vi "Read Multi Eval Meas Magnitude Error Results.vi"(8 "error in (no error)":errorcluster, 9 "Result Type (Current)":i32(ring) items=["Current"=0, "Average"=1, "Maximum"=4], 10 "Instance (1)":T1=1, 11 "VISA resource name":refnum<visa-resource-name>) -> (0 "error out":errorcluster, 1 "Magnitude Error Results":cluster{"Low Window":dbl, "High Window":dbl}[](array[cluster]) {"High Window" format="%^.3e"; "Low Window" format="%^.3e"}, 2 "Reliability":i32, 3 "VISA resource name out":refnum<visa-resource-name>)   [LabVIEW 2020, in "Rohde&Schwarz CMWXP NR FR1 Measurement.lvlib"]
doc: "Returns the values of the magnitude error bar graphs for the OFDM symbols in the measured slot. The results of the current, average and maximum bar graphs can be retrieved.\n\nThere is one pair of magnitude error values per OFDM symbol, for low and high EVM window position respectively.\n\nAttributes:\nRSCMWXPNRFR1M_ATTR_READ_MULTI_EVAL_MEAS_MAGNITUDE_ERROR_CURRENT_RESULTS\nRSCMWXPNRFR1M_ATTR_READ_MULTI_EVAL_MEAS_MAGNITUDE_ERROR_AVERAGE_RESULTS\nRSCMWXPNRFR1M_ATTR_READ_MULTI_EVAL_MEAS_MAGNITUDE_ERROR_MAXIMUM_RESULTS\n\nRemote-control commands:\nREAD:NRSub:MEAS<i>:MEValuation:MERRor:CURRent?\nREAD:NRSub:MEAS<i>:MEValuation:MERRor:AVERage?\nREAD:NRSub:MEAS<i>:MEValuation:MERRor:MAXimum?"
uses:
  <instrlib>/Rohde&Schwarz CMWXP NR FR1 Measurement/Rohde&Schwarz CMWXP NR FR1 Measurement.lvlib
  <instrlib>/Rohde&Schwarz CMWXP NR FR1 Measurement/Private/_Instance.ctl
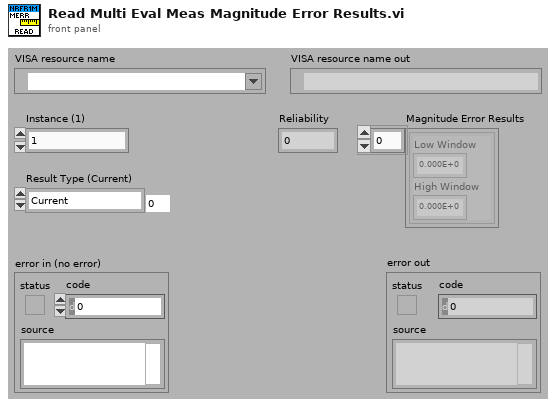
[diagram p1: front panel]
types:
  T1 = typedef "Rohde&Schwarz CMWXP NR FR1 Measurement.lvlib/_Instance.ctl" = i32
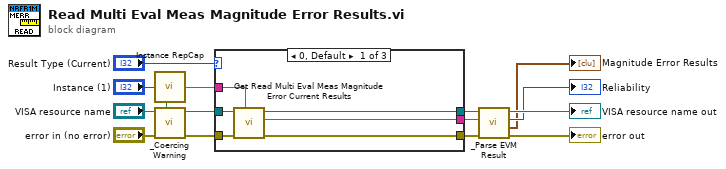
[diagram p0: block diagram]
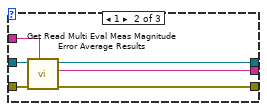
[diagram p2: hidden frame]
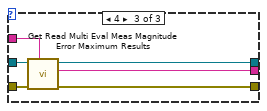
[diagram p3: hidden frame]
diagram:
  n1 = call <instrlib>:"Instance RepCap.vi"("Instance In"="Instance (1)") -> ("In Range?"=w12:bool, "RepCap Identifier Out"=w11:string)  [unwired: 1 in]
  n2 = call <instrlib>:"_Coercing Warning.vi"("In Range?"=w12, "error in (no error)"="error in (no error)", "VISA resource name"="VISA resource name") -> ("error out"=w9:errorcluster, "VISA resource name out"=w10:refnum<visa-resource-name>)  [unwired: 7 in]
  n3 = case shown="0, Default" "Result Type (Current)" {
    tunnel: w11 -> [w21 w27 w33]
    tunnel: w10 -> [w20 w26 w32]
    tunnel: w9 -> [w19 w25 w31]
    tunnel: [w18 w24 w30] -> w5
    tunnel: [w17 w23 w29] -> w6
    tunnel: [w16 w22 w28] -> w7
    frame 0, Default {
      n4 = call "Get Read Multi Eval Meas Magnitude Error Current Results"("Repeated Capabilities"=w21, "error in (no error)"=w19, "instrument handle"=w20) -> ("error out"=w16:errorcluster, "Read Multi Eval Meas Magnitude Error Current Results"=w17:string, "instrument handle out"=w18:refnum<visa-resource-name>)  [unwired: 6 in]
    }
    frame 1 {
      n5 = call "Get Read Multi Eval Meas Magnitude Error Average Results"("Repeated Capabilities"=w27, "error in (no error)"=w25, "instrument handle"=w26) -> ("error out"=w22:errorcluster, "Read Multi Eval Meas Magnitude Error Average Results"=w23:string, "instrument handle out"=w24:refnum<visa-resource-name>)  [unwired: 6 in]
    }
    frame 4 {
      n6 = call "Get Read Multi Eval Meas Magnitude Error Maximum Results"("Repeated Capabilities"=w33, "error in (no error)"=w31, "instrument handle"=w32) -> ("error out"=w28:errorcluster, "Read Multi Eval Meas Magnitude Error Maximum Results"=w29:string, "instrument handle out"=w30:refnum<visa-resource-name>)  [unwired: 6 in]
    }
  }
  n7 = call <instrlib>:"_Parse EVM Result.vi"("error in (no error)"=w7, "Input String"=w6, "VISA resource name"=w5) -> ("error out"=→"error out":errorcluster, "EVM Results"=→"Magnitude Error Results":cluster{"Low Window":dbl, "High Window":dbl}[], "Reliability"=→"Reliability":i32, "VISA resource name out"=→"VISA resource name out":refnum<visa-resource-name>)  [unwired: 5 in]
